vi "Blank Output Stats.vi"(3 "Ch Values in":string[](array[string]), 5 "Indices":i32[](array[numeric])) -> (0 "Ch Values Out":string[](array[string]), 2 "Array Blanked?":bool)   [LabVIEW 2022 SP3]
uses:
  Globals/Meas_global.vi
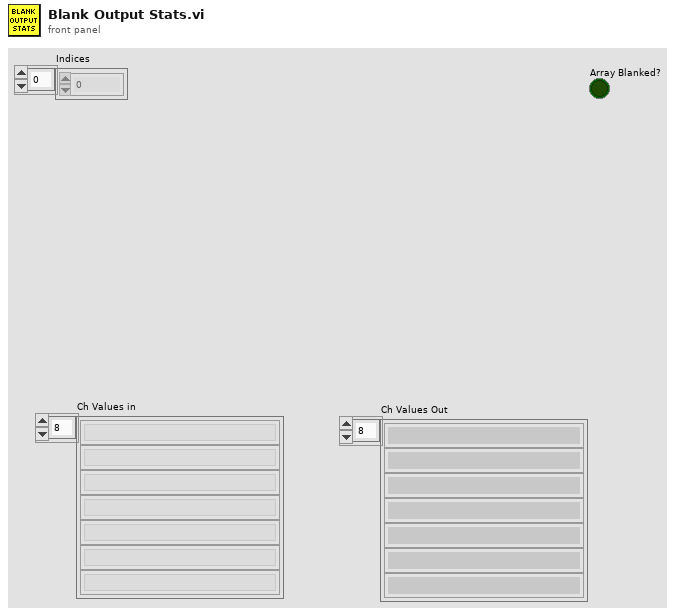
[diagram p1: front panel]
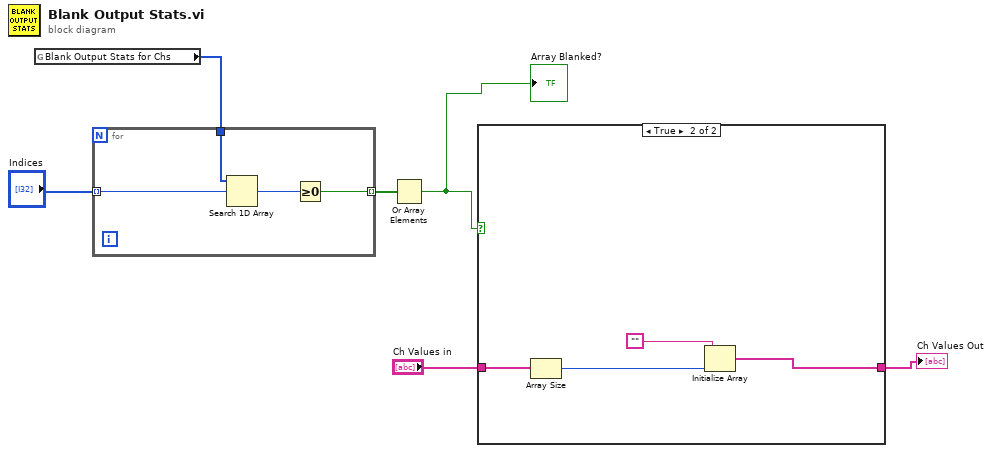
[diagram p0: block diagram]
diagram:
  n1 = global read "Meas_global.vi" "Blank Output Stats for Chs"() -> (w6:i32[])
  n2 = for {
    tunnel: w6 -> [w10]
    tunnel: "Indices" -> [w9] mode=indexing
    tunnel: [w7] -> w4 mode=indexing
    n3 = Search 1D Array(1D array=w10, element=w9) -> (index of element=w8:i32)  [unwired: 1 out]
    n4 = Greater Or Equal To 0?(x=w8) -> (x >= 0?=w7:bool)
  }
  n5 = Or Array Elements(Boolean array=w4) -> (logical OR=w3:bool)
  "Array Blanked?" <- w3
  n6 = case shown="True" w3 {
    tunnel: [w11 w13] -> w2
    tunnel: "Ch Values in" -> [w11 w12]
    frame False {
    }
    frame True {
      n7 = Array Size(array=w12) -> (size(s)=w15:i32)
      n8 = Initialize Array("", w15) -> (w13:string[])
    }
  }
  "Ch Values Out" <- w2
